vi "Run Filter.vi"(8 "error in (no error)":errorcluster, 10 "resource entries in":T1[](array[typedef]) {"FPGA CD Ref" format="%.0x"; "reserver" format="%.0x"}, 11 "RIO Device Filter in":refnum<class "RIO Device Filter.lvclass">) -> (0 "error out":errorcluster, 2 "resource entries out":T1[](array[typedef]) {"FPGA CD Ref" format="%.0x"; "reserver" format="%.0x"})   [LabVIEW 2016, in "FPGA Resource Manager System Defintion.lvlib" / "RIO Device Filter.lvclass"]
uses:
  RIO Device Filter.lvclass
  resource info.ctl
  <vilib>/NI Veristand/Custom Device API/Custom Device Item Ref.ctl
  RIO Device Filter.lvclass/RIO Device Filter.ctl
  <vilib>/NI Veristand/Custom Device API/Get Item Property (String).vi
  <vilib>/NI Veristand/Custom Device API/Custom Device API.lvlib
  FPGA Resource Manager System Defintion.lvlib
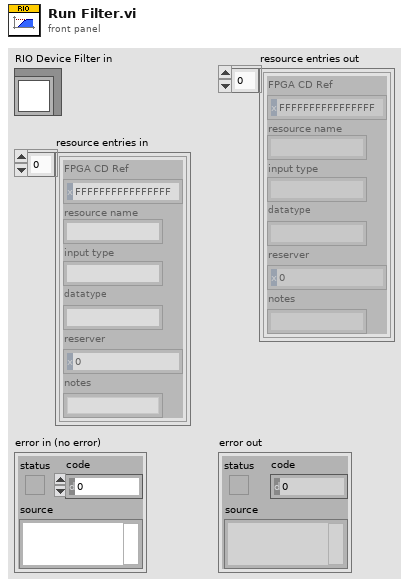
[diagram p1: front panel]
types:
  T1 = typedef "FPGA Resource Manager System Defintion.lvlib/resource info.ctl" = cluster{"FPGA CD Ref":T2, "resource name":string, "input type":string, "datatype":string, "reserver":T2, "notes":string}
  T2 = typedef "Custom Device API.lvlib/Custom Device Item Ref.ctl" = u64
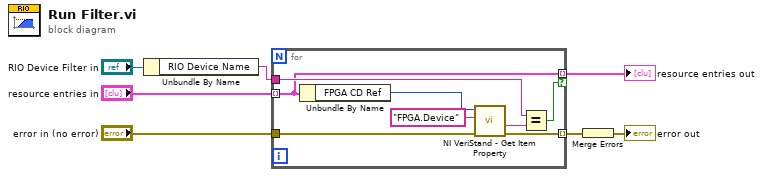
[diagram p0: block diagram]
diagram:
  n1 = Unbundle By Name("RIO Device Filter in") -> ("RIO Device Name"=w5:string)
  n2 = for {
    tunnel: "resource entries in" -> [w12] mode=indexing
    tunnel: w5 -> [w13]
    tunnel: [w12] -> w4 mode=indexing if=w11
    tunnel: "error in (no error)" -> [w10]
    tunnel: [w9] -> w2 mode=indexing
    n3 = Unbundle By Name(w12) -> ("FPGA CD Ref"=w15:T2)
    n4 = call-poly <vilib>:"NI VeriStand - Get Item Property.vi"("error in (no error)"=w10, "Property Name"="FPGA.Device", "Item Ref in"=w15) -> ("error out"=w9:errorcluster, "Value"=w14:string)  [unwired: 5 in, 2 out]
    n5 = Equal?(x=w13, y=w14) -> (x = y?=w11:bool)
  }
  "resource entries out" <- w4
  n6 = Merge Errors(w2) -> (→"error out":errorcluster)
